vi "SaveAutoMeasure.vi"(6 "EN":bool, 7 "Space":T2, 8 "MeasureUp":T1, 9 "MeasureDown":T1, 10 "Measure Name":string(combo)="DL", 11 "MasterPath":path=path "D:/Output") -> (0 "SaveOK":bool, 1 "File path":path, 3 "Folder path":path)   [LabVIEW 2017]
uses:
  <vilib>/Utility/file.llb/Write Delimited Spreadsheet (string).vi
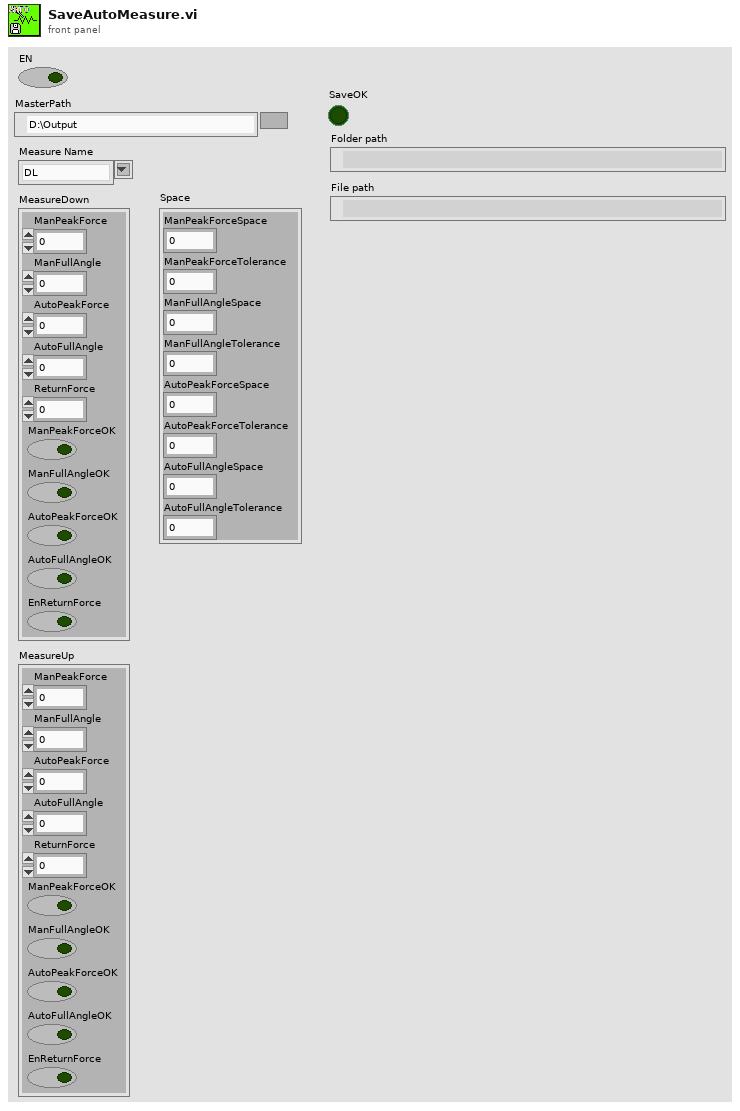
[diagram p1: front panel]
types:
  T1 = cluster{"ManPeakForce":dbl, "ManFullAngle":dbl, "AutoPeakForce":dbl, "AutoFullAngle":dbl, "ReturnForce":dbl, "ManPeakForceOK":bool, "ManFullAngleOK":bool, "AutoPeakForceOK":bool, "AutoFullAngleOK":bool, "EnReturnForce":bool}
  T2 = cluster{"ManPeakForceSpace":dbl, "ManPeakForceTolerance":dbl, "ManFullAngleSpace":dbl, "ManFullAngleTolerance":dbl, "AutoPeakForceSpace":dbl, "AutoPeakForceTolerance":dbl, "AutoFullAngleSpace":dbl, "AutoFullAngleTolerance":dbl}
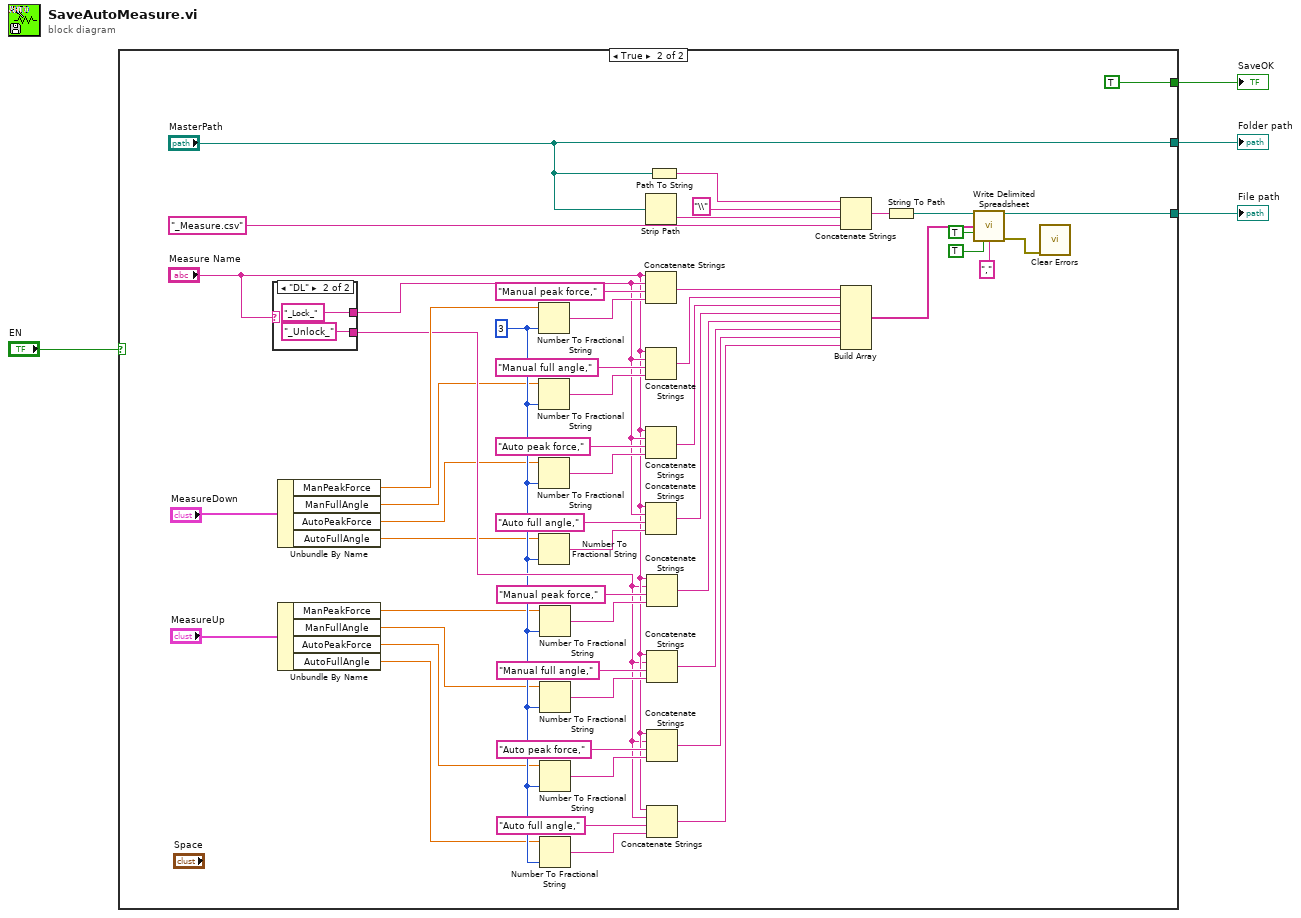
[diagram p0: block diagram]
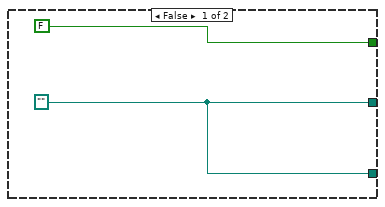
[diagram p2: hidden frame]
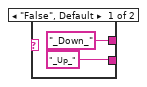
[diagram p3: hidden frame]
diagram:
  n1 = case shown="True" "EN" {
    tunnel: [w5 "MasterPath"] -> w4
    tunnel: [FALSE TRUE] -> w3
    tunnel: [w5 w57] -> w2
    frame False {
      w5 = path ""
    }
    frame True {
      w20 = i16 3 ("precision (6)")
      n2 = case shown="\"DL\"" "Measure Name" {
        tunnel: ["_Down_" ("string") "_Lock_" ("string")] -> w23
        tunnel: ["_Up_" ("string") "_Unlock_" ("string")] -> w21
        frame "False", Default {
        }
        frame "DL" {
        }
      }
      n3 = Unbundle By Name("MeasureDown") -> ("ManPeakForce"=w40:dbl, "ManFullAngle"=w12:dbl, "AutoPeakForce"=w11:dbl, "AutoFullAngle"=w10:dbl)
      n4 = Unbundle By Name("MeasureUp") -> ("ManPeakForce"=w13:dbl, "ManFullAngle"=w9:dbl, "AutoPeakForce"=w8:dbl, "AutoFullAngle"=w7:dbl)
      n5 = Number To Fractional String(number=w40, precision (6)=w20) -> (F-format string=w41:string)  [unwired: 2 in]
      n6 = Number To Fractional String(number=w12, precision (6)=w20) -> (F-format string=w43:string)  [unwired: 2 in]
      n7 = Number To Fractional String(number=w11, precision (6)=w20) -> (F-format string=w46:string)  [unwired: 2 in]
      n8 = Number To Fractional String(number=w10, precision (6)=w20) -> (F-format string=w45:string)  [unwired: 2 in]
      n9 = Number To Fractional String(number=w13, precision (6)=w20) -> (F-format string=w27:string)  [unwired: 2 in]
      n10 = Number To Fractional String(number=w9, precision (6)=w20) -> (F-format string=w26:string)  [unwired: 2 in]
      n11 = Number To Fractional String(number=w8, precision (6)=w20) -> (F-format string=w24:string)  [unwired: 2 in]
      n12 = Number To Fractional String(number=w7, precision (6)=w20) -> (F-format string=w25:string)  [unwired: 2 in]
      n13 = Strip Path(path="MasterPath") -> (name=w33:string)  [unwired: 1 out]
      n14 = Concatenate Strings("Measure Name", w23, "Manual peak force," ("string"), w41) -> (w42:string)
      n15 = Concatenate Strings("Measure Name", w23, "Manual full angle," ("string"), w43) -> (w44:string)
      n16 = Concatenate Strings("Measure Name", w23, "Auto peak force," ("string"), w46) -> (w47:string)
      n17 = Concatenate Strings("Measure Name", w23, "Auto full angle," ("string"), w45) -> (w48:string)
      n18 = Concatenate Strings("Measure Name", w21, "Manual peak force," ("string"), w27) -> (w19:string)
      n19 = Concatenate Strings("Measure Name", w21, "Manual full angle," ("string"), w26) -> (w18:string)
      n20 = Concatenate Strings("Measure Name", w21, "Auto peak force," ("string"), w24) -> (w17:string)
      n21 = Concatenate Strings("Measure Name", w21, "Auto full angle," ("string"), w25) -> (w16:string)
      n22 = Path To String(path="MasterPath") -> (string=w49:string)
      n23 = Concatenate Strings(w49, "\\" ("string"), w33, "_Measure.csv" ("string")) -> (w53:string)
      n24 = Build Array(w42, w44, w47, w48, w19, w18, w17, w16) -> (w35:string[])
      n25 = String To Path(string=w53) -> (path=w52:path)
      n26 = call-poly <vilib>:"Write Delimited Spreadsheet.vi"("file path (dialog if empty)"=w52, "1D data"=w35, "append to file? (new file:F)"=TRUE, "transpose? (no:F)"=TRUE, "delimiter (\\t)"="," ("delimiter (\\t)")) -> ("new file path (Not A Path if cancelled)"=w57:path, "error out"=w51:errorcluster)  [unwired: 9 in]
      n27 = call <vilib>:"Clear Errors.vi"("error in (no error)"=w51) -> ()  [unwired: 5 in, 2 out]
    }
  }
  "Folder path" <- w4
  "SaveOK" <- w3
  "File path" <- w2
